vi "FITS_SaveImageSGL.vi"(1 "Array":sgl[][](array[numeric]) format="%.2f", 2 "Path":path) -> (0 "error out":errorcluster)   [LabVIEW 2016]
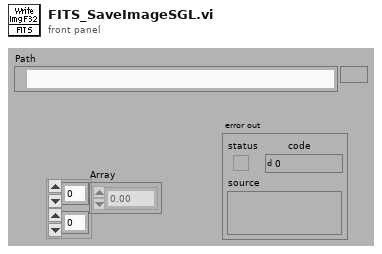
[diagram p1: front panel]
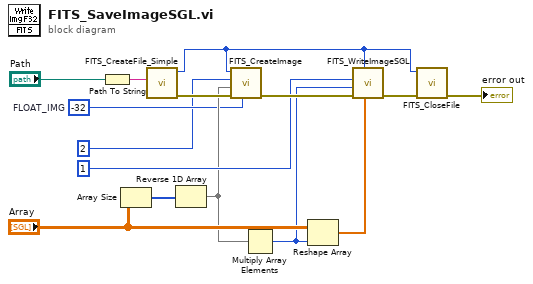
[diagram p0: block diagram]
diagram:
  w2 = -32  # FLOAT_IMG
  n1 = Path To String(path="Path") -> (string=w6:string)
  n2 = Array Size(array="Array") -> (size(s)=w15:i32[])
  n3 = call "FITS_CreateFile_Simple.vi"("filename"=w6) -> ("error out"=w7:errorcluster, "fd"=w4:u64)  [unwired: 1 in, 8 out]
  n4 = Reverse 1D Array(array=w15) -> (reversed array=w3:i32[])
  n5 = call "FITS_CreateImage.vi"("bitpix code"=w2, "error in"=w7, "naxes"=w3, "naxis"=2, "ref in"=w4) -> ("error out"=w10:errorcluster)  [unwired: 6 out]
  n6 = Multiply Array Elements(1:w3) -> (0:w9:i32)
  n7 = Reshape Array("Array", w9) -> (w13:sgl[])
  n8 = call "FITS_WriteImageSGL.vi"("Array"=w13, "ref"=w4, "error in"=w10, "nelem"=w9, "firstel"=1) -> ("error out"=w11:errorcluster)  [unwired: 1 in, 5 out]
  n9 = call "FITS_CloseFile.vi"("error in"=w11, "ref in"=w4) -> ("error out"=→"error out":errorcluster)  [unwired: 1 in, 8 out]
